vi "STAGE+mono+counter_edit14.vi"() -> ()   [LabVIEW 2017]
panel:
  out "XY Graph 2":cluster{dbl[], dbl[]}[](graph)
  out "XY Graph":cluster{dbl[], dbl[]}(graph)
  out "Slide":u8(slide) max=10 step=10 scale=0.0..10.0
  in  "?":enum32{"DELAY", "COUNTER", "MONO", "PLOT"}(tab)
  out "Final time [ps]":dbl
  out "Current time [ps]":dbl
  out "Initial time [ps]":dbl
  in  "Set this as t0":bool
  in  "Axis":i32=1
  in  "Motor ON":bool
  in  "Motor OFF":bool
  out "Current Position [mm]":dbl
  out "Final Position [mm]":dbl
  in  "Data Points":i32=100
  out "Current Point":i32
  in  "Step Size [um]":i32=10
  in  "Target [mm]":dbl format="%.3f"
  in  "Move":bool
  out "Initial position [mm]":dbl
  in  "GPIB address":string="23"
  in  "Count Mode":u16(ring) items=["A,B for Preset T", "A-B for Preset T", "A+B for Preset T", "A for Preset B"]
  in  "Trigger mode":u16(ring) items=["10 MHz"=0, "Input 2"=2, "Input T"=3]
  in  "Channel A Input":u16(ring)=1 items=["10 MHz", "Input 1"]
  in  "Channel B Input":u16(ring)=2 items=["Input 1"=1, "Input 2"=2]
  in  "Number of Measurements\n to take at one point/ Number of Periods":u16=1 min=1 max=2000 step=1
  in  "Time between measurements\n at one point (s)/Dwell Time":dbl=0.002 min=0.002 max=60.0 step=0.001
  in  "gate A mode (CW:0)":i16(slide) scale=0.0..2.0 scale format="%.2f"
  out "Counts":i32
  in  "Integrating time, 10^-7 sec":dbl=10000000.0
  out "Grating #":dbl
  out "Blaze angle":dbl
  out "Grooves/mm":dbl
  out "Mono port":T1(ring)
  out "Time delay":u32=450000 min=1
  in  "Step size":dbl=10.0 min=0.0
  in  "Scan to":i32=4000
  in  "Scan from":i32=2600
  out "Current wavelength":dbl
  in  "?":bool
  in  "Array":dbl[](array[numeric])
  out "Numeric":i32
  out "Numeric 2":i32
  out "Timeout 2":bool
  in  "?":bool
  out "Timeout":bool
  in  "Collect Data!":bool
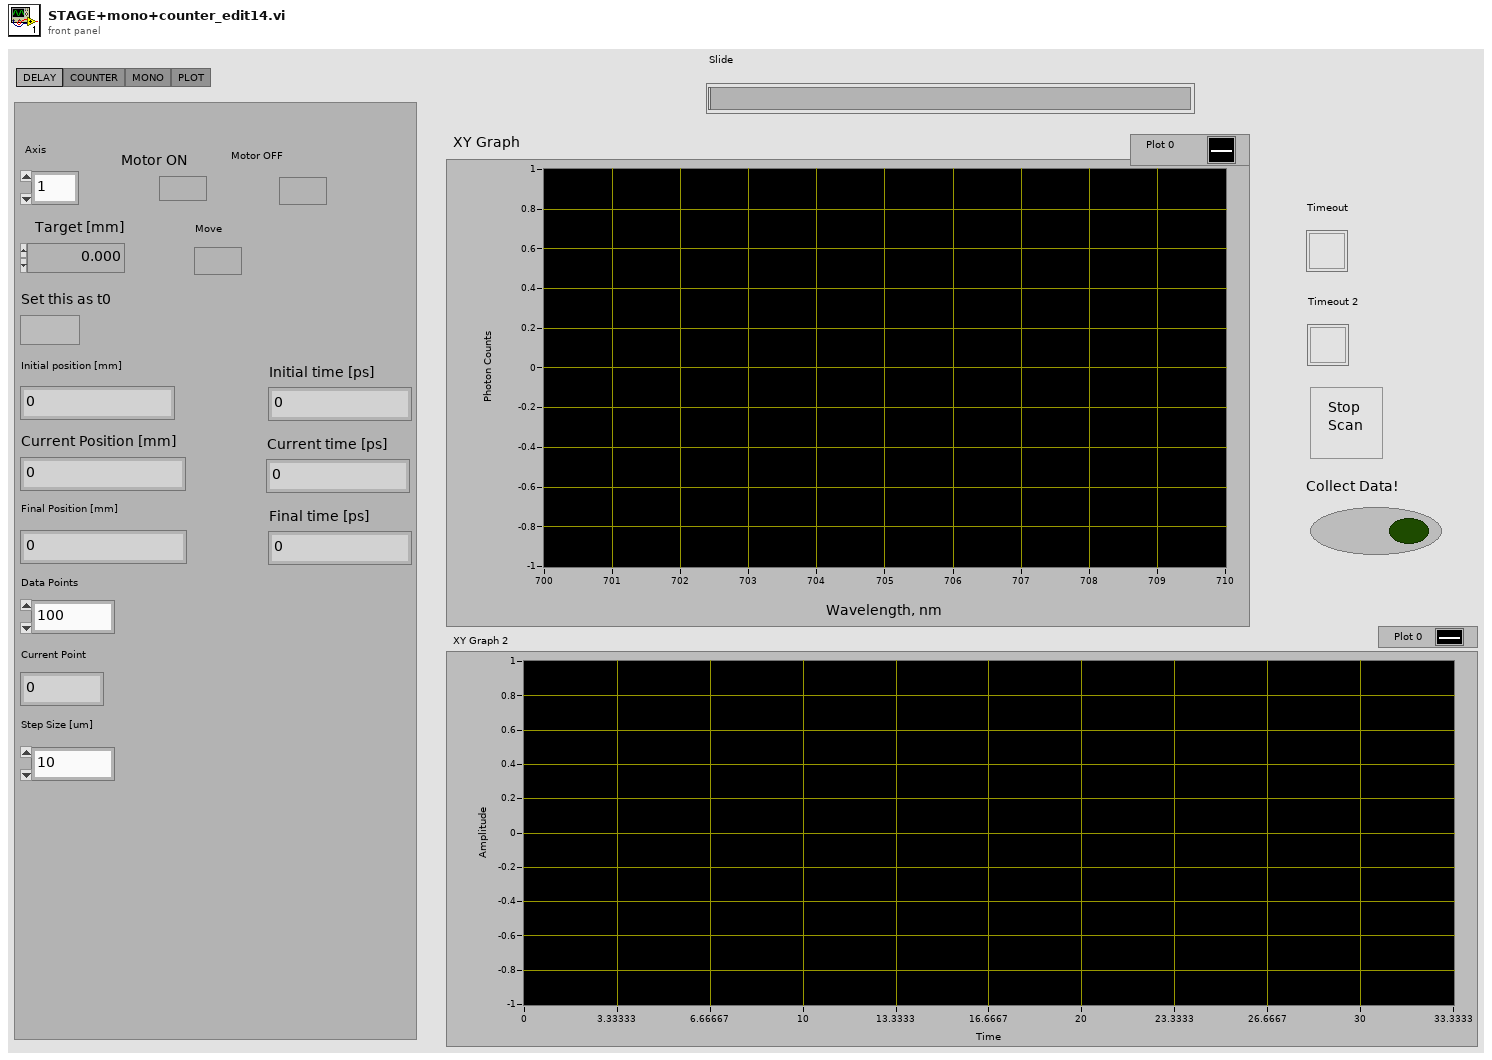
[diagram p1: front panel]
types:
  T1 = enum8{"COM 1", "COM 2", "COM 3", "COM 4", "COM 5", "COM 6", "COM 7", "COM 8", "COM 9"}
  T2 = cluster{"input XON/XOFF":bool, "input HW Handshake":bool, "input alt HW HShk":bool, "output XON/XOFF":bool, "output HW Handshake":bool, "output alt HW HShk":bool, "XOFF byte":u8, "XON byte":u8, "parity error byte":u16}
  T3 = enum16{"no parity", "odd parity", "even parity", "mark parity", "space parity"}
  T4 = cluster{"Y[0]":dbl, "Y[1]":dbl, "Y[2]":dbl, "Y[3]":dbl, "Y[4]":dbl, "Y[5]":dbl, "Y[6]":dbl, "Y[7]":dbl, "Y[8]":dbl}
  T5 = typedef "NI_Matrix.lvlib/RealMatrix.ctl" = dbl[][]
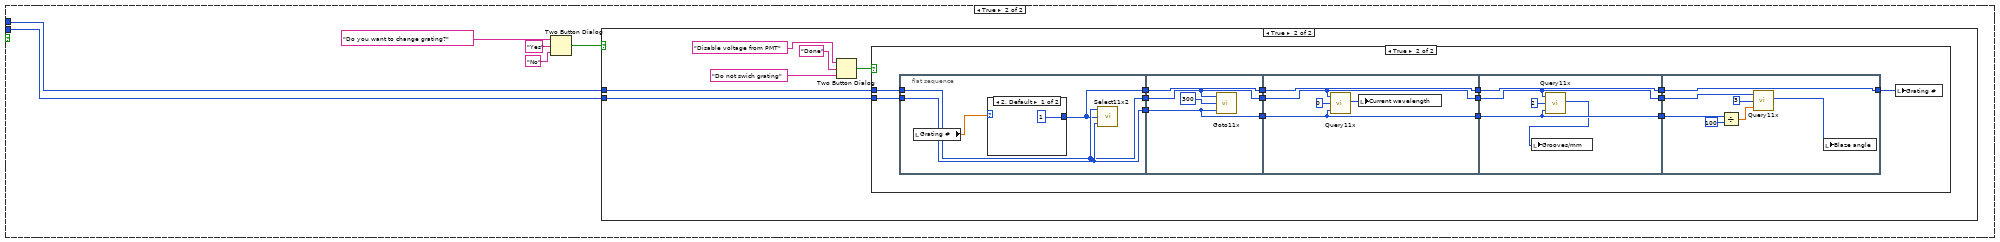
[diagram p2: hidden frame]
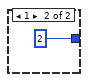
[diagram p5: hidden frame]
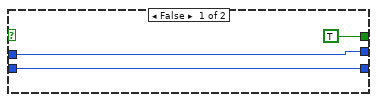
[diagram p6: hidden frame]
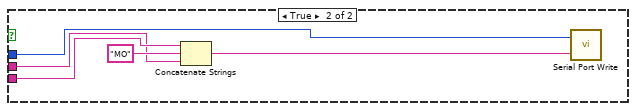
[diagram p7: hidden frame]
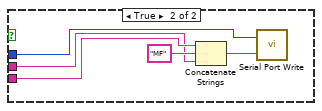
[diagram p8: hidden frame]
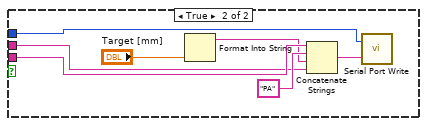
[diagram p9: hidden frame]
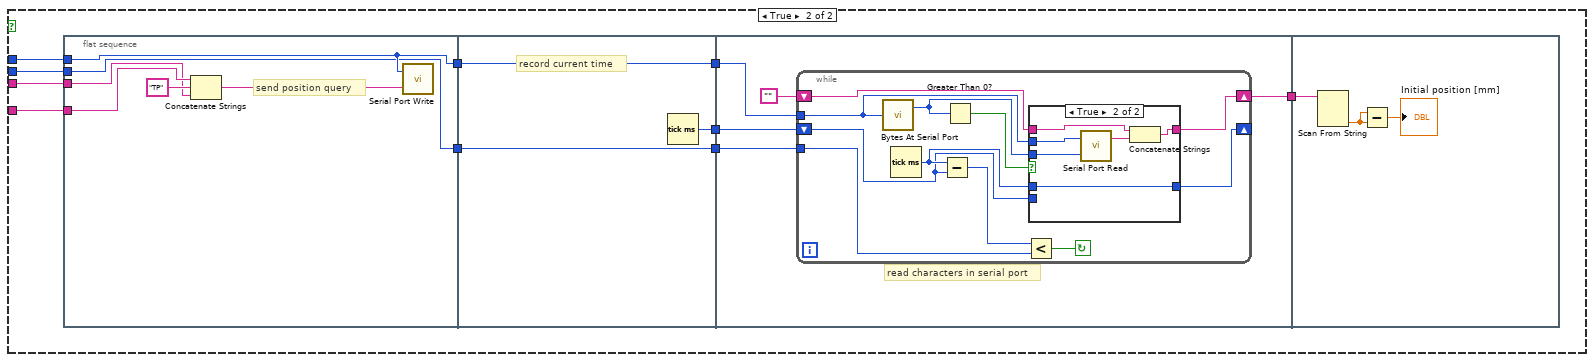
[diagram p10: hidden frame]
diagram:
  (unwired) FALSE
  w48 = u32 19200  # baud rate
  w47 = u16 8  # data bits
  w46 = enum16{"1 bit", "1.5 bits", "2 bits"}."1 bit"  # stop bits
  w50 = T3."no parity"  # parity
  w45 = 4  # 0=COM1 so n=COM(n+1)
  w49 = u16 1024  # buffer size
  n1 = flat-sequence {
    tunnel: ["Data Points"] -> w54
    tunnel: "Axis" -> [w76]
    tunnel: [w68] -> w53
    tunnel: [w76] -> w52
    tunnel: ["Step Size [um]"] -> w14
    tunnel: [w68] -> w13
    tunnel: ["Step Size [um]"] -> w12
    tunnel: ["Data Points"] -> w11
    tunnel: [w68] -> w10
    tunnel: [w67] -> w9
    tunnel: [w68] -> w7
    tunnel: [w67] -> w6
    tunnel: [w70] -> w5
    tunnel: [w60] -> w4
    tunnel: w54 -> [w138]
    tunnel: w53 -> [w137]
    tunnel: w52 -> [w136]
    tunnel: w45 -> [w132]
    tunnel: "GPIB address" -> [w131]
    tunnel: w16 -> [w130]
    tunnel: w15 -> [w129]
    tunnel: "GPIB address" -> [w128]
    tunnel: w14 -> [w115]
    tunnel: w13 -> [w113]
    tunnel: w12 -> [w112]
    tunnel: w11 -> [w110]
    tunnel: w10 -> [w103]
    tunnel: w9 -> [w102]
    tunnel: "Integrating time, 10^-7 sec" -> [w101]
    tunnel: w7 -> [w99]
    tunnel: w6 -> [w98]
    tunnel: w5 -> [w97]
    tunnel: w4 -> [w95]
    frame #0 {
      n2 = while {
        stop <- "Collect Data!" stop-if-true
        n3 = Multiply(x=1, y=1000) -> (x*y=w58:i32)
        n4 = Wait (ms)(milliseconds to wait=w58) -> ()  [unwired: 1 out]
      }
    }
    frame #1 {
      w61 = 1000000000000.0
      w66 = 1000
      w69 = 300000000
      w71 = 1000
      n5 = local read "Initial position [mm]"() -> (w68:dbl)
      n6 = Multiply(x="Step Size [um]", y="Data Points") -> (x*y=w75:i32)
      n7 = Divide(x="Step Size [um]", y=w71) -> (x/y=w70:dbl)
      n8 = Divide(x=w75, y=w71) -> (x/y=w74:dbl)
      n9 = Add(x=w68, y=w74) -> (x+y=w67:dbl)
      "Final Position [mm]" <- w67
      n10 = Divide(x=w68, y=w66) -> (x/y=w64:dbl)
      n11 = Divide(x=w67, y=w66) -> (x/y=w65:dbl)
      n12 = Divide(x=w64, y=w69) -> (x/y=w63:dbl)
      n13 = Divide(x=w65, y=w69) -> (x/y=w62:dbl)
      n14 = Multiply(x=w62, y=w61) -> (x*y=→"Final time [ps]":dbl)
      n15 = Multiply(x=w63, y=w61) -> (x*y=w60:dbl)
      "Initial time [ps]" <- w60
    }
    frame #2 {
      n16 = Increment(x=w110) -> (x+1=w111:i32)
      n17 = Divide(x=w115, y=1000.0) -> (x/y=w89:dbl)
      n18 = for {
        N: w111 -> [_]
        tunnel: w89 -> [w149]
        tunnel: w113 -> [w147]
        tunnel: [w140] -> w109 mode=indexing
        i -> [w148]
        # "distances"
        n19 = Multiply(x=w149, y=w148) -> (x*y=w146:dbl)
        n20 = Add(x=w147, y=w146) -> (x+y=w145:dbl)
        n21 = Divide(x=w145, y=1000) -> (x/y=w139:dbl)
        n22 = Divide(x=w139, y=300000000) -> (x/y=w142:dbl)
        n23 = Multiply(x=w142, y=1000000000000.0) -> (x*y=w140:dbl)
      }
      n24 = Multiply(x="Scan to", y=1) -> (x*y=w96:i32)
      n25 = Multiply(x=1, y="Scan from") -> (x*y=w85:i32)
      n26 = Divide(x=w89, y=1000.0) -> (x/y=w90:dbl)
      n27 = Subtract(x=w96, y=w85) -> (x-y=w123:i32)
      n28 = local read "Numeric 2"() -> (w78:i32)
      n29 = local read "Numeric"() -> (w77:i32)
      n30 = Divide(x=w123, y="Step size") -> (x/y=w122:dbl)
      n31 = Divide(x=w90, y=300000000) -> (x/y=w92:dbl)
      n32 = Multiply(x=w92, y=1000000000000.0) -> (x*y=w88:dbl)
      n33 = Build Array(w95) -> (w82:dbl[])
      n34 = Round Toward -Infinity(1:w122) -> (0:w121:dbl)
      n35 = Concatenate Strings("\r", "\n") -> (w133:string)
      n36 = Initialize Array(0, w77, w78) -> (w80:i32[][])
      n37 = Increment(x=w121) -> (x+1=w84:dbl)
      n38 = for {
        N: w138 -> [w197]
        tunnel: w137 -> [w224]
        tunnel: w112 -> [w220]
        tunnel: w136 -> [w217]
        tunnel: w133 -> [w214]
        tunnel: w132 -> [w215]
        tunnel: w131 -> [w213]
        tunnel: w130 -> [w210]
        tunnel: w129 -> [w212]
        tunnel: w128 -> [w211]
        tunnel: [w162] -> w118 mode=indexing
        tunnel: w85 -> [w205]
        tunnel: "Step size" -> [w204]
        tunnel: w121 -> [w203]
        tunnel: w103 -> [_]
        tunnel: w102 -> [_]
        tunnel: w101 -> [w202]
        tunnel: "Scan to" -> [w201]
        tunnel: "Scan from" -> [w200]
        tunnel: "Step size" -> [w171]
        tunnel: w99 -> [w192]
        tunnel: w98 -> [w190]
        tunnel: w97 -> [w193]
        tunnel: w88 -> [w180]
        shift-right: [w164] -> _
        shift-left: w82 -> [w174]
        shift-right: [w163] -> _
        shift-left: dbl[] [] ("Y") -> [w169]
        tunnel: w95 -> [w198]
        tunnel: "Scan from" -> [w172]
        tunnel: "Step size" -> [w173]
        shift-right: [w161] -> _
        shift-left: w82 -> [w167]
        shift-right: [w159] -> _
        shift-left: w80 -> [w158]
        i -> [w179]
        w191 = 1000
        w194 = 300000000
        n39 = To Time Stamp(1:w205) -> ()  [unwired: 1 out]
        n40 = property on="Slide" class="Slide (strict)"("Scale.Increment"=1, "Scale.Maximum"=w197, "Scale.Minimum"=0) -> ()  [unwired: 2 in, 2 out]
        n41 = stacked-sequence {
          tunnel: w210 -> [w344]
          tunnel: w211 -> [_]
          frame #0 {
            n42 = call <vilib>:"Close Serial Driver.vi"("port number"=w344) -> ()  [unwired: 1 out]
            n43 = GPIB Misc(0:"loc 23" ("command string")) -> ()  [unwired: 1 in, 3 out]
          }
        }
        n44 = Multiply(x=w180, y=w179) -> (x*y=w199:dbl)
        n45 = Divide(x=w192, y=w191) -> (x/y=w188:dbl)
        n46 = Divide(x=w193, y=w191) -> (x/y=w189:dbl)
        n47 = Divide(x=w190, y=w191) -> (x/y=w187:dbl)
        n48 = Number To Decimal String(number=w202) -> (decimal integer string=w208:string)  [unwired: 1 in]
        n49 = Build Array(w172) -> (w176:i32[])
        n50 = Add(x=1, y=w179) -> (x+y=→"Slide":i32)
        n51 = Divide(x=w220, y=1000) -> (x/y=w219:dbl)
        n52 = Divide(x=w188, y=w194) -> (x/y=w182:dbl)
        n53 = Divide(x=w189, y=w194) -> (x/y=w183:dbl)
        n54 = Divide(x=w187, y=w194) -> (x/y=w181:dbl)
        n55 = Add(x=w198, y=w199) -> (x+y=w168:dbl)
        n56 = Concatenate Strings("CP 2,", w208) -> (w206:string)
        n57 = flat-sequence {
          tunnel: w213 -> [w238]
          tunnel: w212 -> [w237]
          tunnel: w210 -> [w236]
          tunnel: w205 -> [w235]
          tunnel: w204 -> [w234]
          tunnel: w203 -> [w233]
          tunnel: w201 -> [w232]
          tunnel: w200 -> [w231]
          tunnel: w176 -> [w230]
          tunnel: dbl[] [] ("Y") -> [w229]
          tunnel: w173 -> [w228]
          tunnel: w172 -> [w227]
          tunnel: w171 -> [w226]
          tunnel: [w225] -> w170
          tunnel: w170 -> [w298]
          tunnel: w169 -> [w305]
          tunnel: [w298] -> w166
          tunnel: w165 -> [w302]
          tunnel: [w300] -> w164
          tunnel: [w299] -> w163
          tunnel: [w298] -> w162
          tunnel: w166 -> [w314]
          tunnel: [w307] -> w161
          tunnel: w160 -> [w308]
          tunnel: w158 -> [w311]
          tunnel: [w309] -> w159
          frame #0 {
            # "step size"
            n58 = while {
              tunnel: w236 -> [w270]
              tunnel: w237 -> [w269]
              tunnel: w238 -> [w265]
              tunnel: w235 -> [w263]
              tunnel: w234 -> [w262]
              tunnel: w233 -> [w261]
              tunnel: w232 -> [w245]
              tunnel: w231 -> [w246]
              tunnel: w226 -> [w247]
              tunnel: w228 -> [w259]
              shift-right: [w254] -> w225
              shift-left: w229 -> [w253]
              shift-right: [w248] -> _
              shift-left: w230 -> [w257]
              tunnel: w227 -> [w251]
              i -> [w260]
              stop <- w268 stop-if-true
              n59 = property on="XY Graph" class="XYGraph (strict)"("XScale.Increment"=w247, "XScale.Maximum"=w245, "XScale.Minimum"=w246) -> ()  [unwired: 2 in, 2 out]
              n60 = Multiply(x=w260, y=w262) -> (x*y=w271:dbl)
              n61 = Multiply(x=w260, y=w259) -> (x*y=w258:dbl)
              n62 = Greater Or Equal?(x=w260, y=w261) -> (x >= y?=w266:bool)
              n63 = Add(x=w258, y=w251) -> (x+y=w256:dbl)
              n64 = Add(x=w271, y=w263) -> (x+y=w264:dbl)
              n65 = Or(x="?", y=w266) -> (x .or. y?=w268:bool)
              n66 = flat-sequence {
                tunnel: w264 -> [w276]
                tunnel: w270 -> [w275]
                tunnel: w269 -> [w274]
                tunnel: w265 -> [w272]
                tunnel: [w275] -> w244
                tunnel: [w274] -> w243
                tunnel: [w272] -> w242
                tunnel: w244 -> [w283]
                tunnel: w243 -> [w282]
                tunnel: w242 -> [w277]
                tunnel: [w277] -> w241
                tunnel: w241 -> [w285]
                tunnel: [w285] -> w240
                tunnel: w240 -> [w286]
                tunnel: [w286] -> w239
                tunnel: [w292] -> w250
                tunnel: w239 -> [w293]
                frame #0 {
                  n67 = call "Goto11x.vi"("time delay"=w274, "WAVELENGTH"=w276, "port number"=w275) -> ("timeout"=w273:bool)  [unwired: 2 out]
                  n68 = local write "Timeout 2"(w273) -> ()
                }
                frame #1 {
                  # "set counter time in 10^-7 seconds in CW"
                  n69 = call "Query11x.vi"("port number"=w283, "QUERY"=0, "time delay"=w282) -> ("timeout"=w281:bool, "STATUS MESSAGE"=w280:u16)  [unwired: 2 out]
                  n70 = local write "Timeout 2"(w281) -> ()
                  n71 = Divide(x=w280, y=10) -> (x/y=w279:dbl)
                  n72 = local write "Current wavelength"(w279) -> ()
                }
                frame #2 {
                  n73 = call "Start.vi"("GPIB Address"=w285) -> ()  [unwired: 9 in]
                }
                frame #3 {
                  # "Wait for Scan to Finish"
                  n74 = for {
                    N: 1 -> [_]
                    tunnel: w286 -> [w288]
                    n75 = while {
                      tunnel: w288 -> [w289]
                      stop <- w291 stop-if-true
                      n76 = call "ScanDone.vi"("Wait (ms)"=1000, "GPIB Address"=w289) -> ("Scan Finished?"=w291:bool)
                    }
                  }
                }
                frame #4 {
                  n77 = call "Read Data.vi"("Channel Number"=0, "GPIB Address"=w293, "Number of Datapoints"=1) -> ("Data"=w294:i32[])
                  n78 = Index Array(array=w294, index=0) -> (element=w292:i32)
                  "Counts" <- w292
                }
              }
              n79 = Build Array (concatenate)(w257, w256) -> (w255:dbl[])
              n80 = Build Array (concatenate)(w253, w250) -> (w252:dbl[])
              n81 = Bundle(w255, w252) -> (w249:cluster{dbl[], dbl[]})  [unwired: 1 in]
              "XY Graph" <- w249
              n82 = Unbundle(w249) -> (w248:dbl[], w254:dbl[])
            }
          }
          frame #1 {
            n83 = Array To Cluster(array=w298) -> (cluster=w306:T4)
            n84 = Unbundle By Name(w306) -> ("Y[5]"=w304:dbl)  [unwired: 10 out]
            n85 = Build Array (concatenate)(w305, w304) -> (w303:dbl[])
            n86 = Bundle(w302, w303) -> (w301:cluster{dbl[], dbl[]})  [unwired: 1 in]
            n87 = Unbundle(w301) -> (w300:dbl[], w299:dbl[])
          }
          frame #2 {
            n88 = Array Size(array="Array") -> (size(s)=w312:i32)
            n89 = flat-sequence {
              tunnel: w314 -> [w319]
              tunnel: "Array" -> [w318]
              tunnel: w312 -> [w317]
              tunnel: [w315] -> w310
              tunnel: w311 -> [w336]
              tunnel: w310 -> [w335]
              tunnel: [w333] -> w309
              tunnel: w308 -> [w332]
              tunnel: [w331] -> w307
              frame #0 {
                n90 = for {
                  N: w317 -> [w321]
                  tunnel: w318 -> [w329]
                  tunnel: w319 -> [w323]
                  tunnel: [w320] -> w316
                  i -> [w328]
                  n91 = local read "Scan from"() -> (w326:i32)
                  n92 = Index Array(array=w329, index=w328) -> (element=w327:dbl)
                  n93 = local read "Step size"() -> (w324:dbl)
                  n94 = Subtract(x=w327, y=w326) -> (x-y=w325:dbl)
                  n95 = Divide(x=w325, y=w324) -> (x/y=w322:dbl)
                  n96 = Index Array(array=w323, index=w322) -> (element=w320:dbl)
                  "Numeric" <- w321
                }
                n97 = Build Array(w316) -> (w315:dbl[])
              }
              frame #1 {
                n98 = local read "Numeric"() -> (w334:i32)
                n99 = Build Array (concatenate)(w336, w335) -> (w333:dbl[][])
                n100 = for {
                  N: w334 -> [_]
                  tunnel: w333 -> [w342]
                  tunnel: w332 -> [w340]
                  tunnel: [w339] -> w331
                  tunnel: [w337] -> w330 mode=indexing
                  i -> [w341]
                  n101 = Index Array(array=w342, index (row)=w341) -> (element=w338:dbl[])  [unwired: 1 in]
                  n102 = Bundle(w340, w338) -> (w337:cluster{dbl[], dbl[]})  [unwired: 1 in]
                  n103 = Unbundle(w337) -> (w339:dbl[])  [unwired: 1 out]
                }
                "XY Graph 2" <- w330
              }
            }
          }
        }
        n104 = Multiply(x=w219, y=w179) -> (x*y=w223:dbl)
        n105 = Multiply(x=w182, y=1000000000000.0) -> (x*y=w156:dbl)
        n106 = Multiply(x=w183, y=1000000000000.0) -> (x*y=w157:dbl)
        n107 = Multiply(x=w181, y=1000000000000.0) -> (x*y=w155:dbl)
        n108 = Build Array (concatenate)(w167, w168) -> (w160:dbl[])
        n109 = Build Array (concatenate)(w174, w168) -> (w165:dbl[])
        n110 = property on="XY Graph 2" class="XYGraph (strict)"("XScale.Increment"=w157, "XScale.Maximum"=w155, "XScale.Minimum"=w156) -> ()  [unwired: 2 in, 2 out]
        n111 = Add(x=w224, y=w223) -> (x+y=w222:dbl)
        n112 = Format Into String(w217) -> (resulting string=w216:string)  [unwired: 3 in, 1 out]
        n113 = GPIB Write(0:w213, 1:w206, 2:i16 5 ("mode (0)")) -> ()  [unwired: 2 in, 2 out]
        n114 = flat-sequence {
          tunnel: w222 -> [w347]
          tunnel: [w347] -> w218
          tunnel: w214 -> [w349]
          tunnel: w216 -> [w348]
          tunnel: w215 -> [w345]
          tunnel: w218 -> [w358]
          frame #0 {
            n115 = Format Into String(w347) -> (resulting string=w346:string)  [unwired: 3 in, 1 out]
            n116 = Wait (ms)(milliseconds to wait=u32 100) -> ()  [unwired: 1 out]
            n117 = Concatenate Strings(w348, "PA" ("Substring"), w346, w349) -> (w351:string)
            n118 = call <vilib>:"Serial Port Write.vi"("string to write"=w351, "port number"=w345) -> ()  [unwired: 1 out]
          }
          frame #1 {
            n119 = Divide(x=w358, y=1000) -> (x/y=w356:dbl)
            n120 = Wait (ms)(milliseconds to wait=u32 1000) -> ()  [unwired: 1 out]
            n121 = Divide(x=w356, y=300000000) -> (x/y=w355:dbl)
            n122 = Multiply(x=w355, y=1000000000000.0) -> (x*y=→"Current time [ps]":dbl)
            "Current Position [mm]" <- w358
          }
        }
        "Current Point" <- w179
        "Numeric 2" <- w197
      }
      n123 = for {
        N: w84 -> [_]
        tunnel: "Step size" -> [w154]
        tunnel: w85 -> [w152]
        tunnel: [w150] -> w83 mode=indexing
        i -> [w153]
        # "wavelengths"
        n124 = Multiply(x=w154, y=w153) -> (x*y=w151:dbl)
        n125 = Add(x=w152, y=w151) -> (x+y=w150:dbl)
      }
      n126 = Build Array (concatenate)(0, w109) -> (w106:dbl[])
      n127 = Build Array(w83) -> (w119:dbl[][])
      n128 = Transpose Matrix(1:w118) -> (0:w116:dbl[][])
      n129 = Transpose Matrix(1:w119) -> (0:w117:dbl[][])
      n130 = Build Array (concatenate)(w117, w116) -> (w105:T5)
      n131 = Insert Into Array(array=w105, index (row)=0, new element=w106) -> (w104:T5)  [unwired: 1 in]
      n132 = Array To Spreadsheet String(delimiter (Tab)=",", array=w104, 3:"%f" ("format string")) -> (spreadsheet string=w120:string)
      n133 = Write to Text File(text=w120) -> ()  [unwired: 3 in, 3 out]
    }
  }
  n134 = flat-sequence {
    tunnel: [w362] -> w30
    tunnel: [w361] -> w29
    frame #0 {
      n135 = call "CM Com Read ini.vi"() -> ("Mono port"=w361:T1, "time delay1"=w362:u32)  [unwired: 7 in]
    }
  }
  n136 = call <vilib>:"Serial Port Init.vi"("flow control etc."=T2 {"input XON/XOFF"=FALSE, "input HW Handshake"=FALSE, "input alt HW HShk"=FALSE, "output XON/XOFF"=FALSE, "output HW Handshake"=FALSE, "output alt HW HShk"=FALSE, "XOFF byte"=13, "XON byte"=11, "parity error byte"=0}, "parity"=w50, "buffer size"=w49, "stop bits"=w46, "data bits"=w47, "baud rate"=w48, "port number"=w45) -> ("error code"=w44:i32)
  n137 = call "CM Serial Port Setup.vi"("COM port"=w29, "time delay"=w30) -> ("time delay1"=w25:u32, "DK port Out"=w26:T1, "error code"=w28:i32)  [unwired: 7 in]
  n138 = Concatenate Strings("\r", "\n") -> (w40:string)
  n139 = Equal To 0?(x=w28) -> (x = 0?=w27:bool)
  n140 = while {
    tunnel: w45 -> [w377]
    tunnel: w40 -> [w378]
    tunnel: w44 -> [_]
    tunnel: "Axis" -> [w375]
    stop <- TRUE continue-if-true
    w376 = u32 200  # timeout
    n141 = Format Into String(w375) -> (resulting string=w379:string)  [unwired: 3 in, 1 out]
    n142 = flat-sequence {
      tunnel: w379 -> [w384]
      tunnel: w378 -> [w383]
      tunnel: w377 -> [w385]
      tunnel: w376 -> [w382]
      tunnel: [w384] -> w374
      tunnel: [w383] -> w373
      tunnel: [w385] -> w372
      tunnel: [w382] -> w371
      tunnel: w374 -> [w395]
      tunnel: w373 -> [w394]
      tunnel: w372 -> [w396]
      tunnel: w371 -> [w392]
      tunnel: [w395] -> w370
      tunnel: [w394] -> w369
      tunnel: [w396] -> w368
      tunnel: [w392] -> w367
      tunnel: w370 -> [w405]
      tunnel: w369 -> [w404]
      tunnel: w368 -> [w406]
      tunnel: w367 -> [w402]
      tunnel: [w405] -> w366
      tunnel: [w404] -> w365
      tunnel: [w406] -> w364
      tunnel: [w402] -> w363
      tunnel: w366 -> [w418]
      tunnel: w365 -> [w415]
      tunnel: w364 -> [w417]
      tunnel: w363 -> [w416]
      frame #0 {
        n143 = case shown="False" "Motor ON" {
          tunnel: w385 -> [_ w391]
          tunnel: w384 -> [_ w388]
          tunnel: w383 -> [_ w387]
          frame False {
          }
          frame True {
            n144 = Concatenate Strings(w388, "MO" ("Substring"), w387) -> (w389:string)
            n145 = call <vilib>:"Serial Port Write.vi"("string to write"=w389, "port number"=w391) -> ()  [unwired: 1 out]
          }
        }
      }
      frame #1 {
        n146 = case shown="False" "Motor OFF" {
          tunnel: w396 -> [_ w401]
          tunnel: w395 -> [_ w398]
          tunnel: w394 -> [_ w397]
          frame False {
          }
          frame True {
            n147 = Concatenate Strings(w398, "MF" ("Substring"), w397) -> (w399:string)
            n148 = call <vilib>:"Serial Port Write.vi"("string to write"=w399, "port number"=w401) -> ()  [unwired: 1 out]
          }
        }
      }
      frame #2 {
        n149 = case shown="False" "Move" {
          tunnel: w406 -> [_ w413]
          tunnel: w405 -> [_ w410]
          tunnel: w404 -> [_ w409]
          frame False {
          }
          frame True {
            n150 = Format Into String("Target [mm]") -> (resulting string=w407:string)  [unwired: 3 in, 1 out]
            n151 = Concatenate Strings(w410, "PA" ("Substring"), w407, w409) -> (w411:string)
            n152 = call <vilib>:"Serial Port Write.vi"("string to write"=w411, "port number"=w413) -> ()  [unwired: 1 out]
          }
        }
      }
      frame #3 {
        n153 = case shown="False" "Set this as t0" {
          tunnel: w418 -> [_ w428]
          tunnel: w417 -> [_ w427]
          tunnel: w416 -> [_ w426]
          tunnel: w415 -> [_ w425]
          frame False {
          }
          frame True {
            n154 = flat-sequence {
              tunnel: w428 -> [w432]
              tunnel: w427 -> [w431]
              tunnel: [w431] -> w424
              tunnel: w426 -> [w429]
              tunnel: [w429] -> w423
              tunnel: w425 -> [w430]
              tunnel: w424 -> [w436]
              tunnel: [w436] -> w422
              tunnel: w423 -> [w435]
              tunnel: [w435] -> w421
              tunnel: [w437] -> w420
              tunnel: w422 -> [w442]
              tunnel: w421 -> [w440]
              tunnel: w420 -> [w439]
              tunnel: [w438] -> w419
              tunnel: w419 -> [w464]
              frame #0 {
                # "send position query"
                n155 = Concatenate Strings(w432, "TP" ("Substring"), w430) -> (w433:string)
                n156 = call <vilib>:"Serial Port Write.vi"("string to write"=w433, "port number"=w431) -> ()  [unwired: 1 out]
              }
              frame #1 {
                # "record current time"
                n157 = Tick Count (ms)() -> (millisecond timer value=w437:u32)
              }
              frame #2 {
                # "read characters in serial port"
                n158 = while {
                  shift-left: w439 -> [w443]
                  shift-right: [w444] -> _
                  tunnel: w440 -> [w447]
                  shift-left: "" -> [w450]
                  shift-right: [w449] -> w438
                  tunnel: w442 -> [w451]
                  stop <- w446 continue-if-true
                  n159 = call <vilib>:"Bytes At Serial Port.vi"("port number"=w451) -> ("byte count"=w452:u32)  [unwired: 1 out]
                  n160 = Tick Count (ms)() -> (millisecond timer value=w445:u32)
                  n161 = Subtract(x=w445, y=w443) -> (x-y=w448:u32)
                  n162 = Greater Than 0?(x=w452) -> (x > 0?=w453:bool)
                  n163 = Less?(x=w448, y=w447) -> (x < y?=w446:bool)
                  n164 = case shown="True" w453 {
                    tunnel: w452 -> [_ w461]
                    tunnel: w451 -> [_ w460]
                    tunnel: w450 -> [w455 w458]
                    tunnel: [w455 w457] -> w449
                    tunnel: [w454 w456] -> w444
                    tunnel: w445 -> [_ w456]
                    tunnel: w443 -> [w454 _]
                    frame False {
                    }
                    frame True {
                      n165 = call <vilib>:"Serial Port Read.vi"("requested byte count"=w461, "port number"=w460) -> ("string read"=w459:string)  [unwired: 1 out]
                      n166 = Concatenate Strings(w458, w459) -> (w457:string)
                    }
                  }
                }
              }
              frame #3 {
                n167 = Scan From String(input string=w464) -> (output 1=w462:dbl)  [unwired: 4 in, 3 out]
                n168 = Subtract(x=w462, y=w462) -> (x-y=→"Initial position [mm]":dbl)
              }
            }
          }
        }
      }
    }
    n169 = Wait Until Next ms Multiple(millisecond multiple=u32 50) -> ()  [unwired: 1 out]
  }
  n170 = case shown="True" w27 {
    tunnel: w26 -> [w467 w470]
    tunnel: w25 -> [w466 w469]
    tunnel: [w467 w470] -> w16
    tunnel: [w466 w469] -> w15
    tunnel: [TRUE FALSE] -> w24
    frame False {
    }
    frame True {
      n171 = call "CM Com Write ini.vi"("time delay1"=w470, "Mono port"=w469) -> ()  [unwired: 7 in]
      n172 = local write "Mono port"(w470) -> ()
      n173 = local write "Time delay"(w469) -> ()
    }
  }
  n174 = flat-sequence {
    tunnel: w15 -> [w476]
    tunnel: [w476] -> w39
    tunnel: w16 -> [w478]
    tunnel: [w478] -> w38
    tunnel: w24 -> [w474]
    tunnel: [w474] -> w37
    tunnel: w39 -> [w482]
    tunnel: [w482] -> w36
    tunnel: w38 -> [w483]
    tunnel: [w483] -> w35
    tunnel: w37 -> [w480]
    tunnel: [w480] -> w34
    tunnel: w36 -> [w491]
    tunnel: [w491] -> w33
    tunnel: w35 -> [w488]
    tunnel: [w488] -> w32
    tunnel: w34 -> [w486]
    tunnel: [w486] -> w31
    tunnel: w33 -> [w494]
    tunnel: w32 -> [w493]
    tunnel: w31 -> [_]
    frame #0 {
      n175 = call "Query11x.vi"("port number"=w478, "QUERY"=u16 0, "time delay"=w476) -> ("timeout"=w475:bool, "STATUS MESSAGE"=w473:u16)  [unwired: 2 out]
      n176 = local write "Timeout"(w475) -> ()
      n177 = Divide(x=w473, y=10 ("Numeric")) -> (x/y=→"Current wavelength":dbl)
    }
    frame #1 {
      n178 = call "Query11x.vi"("port number"=w483, "QUERY"=u16 2, "time delay"=w482) -> ("timeout"=w481:bool, "STATUS MESSAGE"=→"Grooves/mm":u16)  [unwired: 2 out]
      n179 = local write "Timeout"(w481) -> ()
    }
    frame #2 {
      n180 = Divide(x=w491, y=i16 100 ("device (1)")) -> (x/y=w489:dbl)
      n181 = call "Query11x.vi"("port number"=w488, "QUERY"=u16 3, "time delay"=w489) -> ("timeout"=w487:bool, "STATUS MESSAGE"=→"Blaze angle":u16)  [unwired: 2 out]
      n182 = local write "Timeout"(w487) -> ()
    }
    frame #3 {
      n183 = Divide(x=w494, y=i16 100 ("device (1)")) -> (x/y=w497:dbl)
      n184 = call "Query11x.vi"("port number"=w493, "QUERY"=u16 4, "time delay"=w497) -> ("timeout"=w496:bool, "STATUS MESSAGE"=→"Grating #":u16)  [unwired: 2 out]
      n185 = local write "Timeout"(w496) -> ()
    }
  }
  n186 = case shown="False" "?" {
    tunnel: w15 -> [_ w501]
    tunnel: w16 -> [_ w500]
    frame False {
    }
    frame True {
      n187 = Two Button Dialog(message="Do you want to change grating?", 1:"No" ("F button name (\"Cancel\")"), 2:"Yes" ("T button name (\"OK\")")) -> (T button?=w502:bool)
      n188 = case shown="True" w502 {
        tunnel: w501 -> [_ w507]
        tunnel: w500 -> [_ w506]
        frame False {
        }
        frame True {
          n189 = Two Button Dialog(message="Disable voltage from PMT", 1:"Do not swich grating" ("F button name (\"Cancel\")"), 2:"Done" ("T button name (\"OK\")")) -> (T button?=w508:bool)
          n190 = case shown="True" w508 {
            tunnel: w507 -> [_ w526]
            tunnel: w506 -> [_ w525]
            frame False {
            }
            frame True {
              n191 = flat-sequence {
                tunnel: w526 -> [w530]
                tunnel: [w530] -> w523
                tunnel: w525 -> [w529]
                tunnel: [w529] -> w522
                tunnel: [w527] -> w521
                tunnel: w523 -> [w534]
                tunnel: [w534] -> w520
                tunnel: w522 -> [w535]
                tunnel: [w535] -> w519
                tunnel: w521 -> [w533]
                tunnel: [w533] -> w518
                tunnel: w520 -> [w541]
                tunnel: [w541] -> w517
                tunnel: w519 -> [w540]
                tunnel: [w540] -> w516
                tunnel: w518 -> [w538]
                tunnel: [w538] -> w515
                tunnel: w517 -> [w544]
                tunnel: [w544] -> w514
                tunnel: w516 -> [w545]
                tunnel: [w545] -> w513
                tunnel: w515 -> [w543]
                tunnel: [w543] -> w512
                tunnel: w514 -> [w549]
                tunnel: w513 -> [w550]
                tunnel: [w548] -> w524
                tunnel: w512 -> [w548]
                frame #0 {
                  n192 = local read "Grating #"() -> (w528:dbl)
                  n193 = case shown="2, Default" w528 {
                    tunnel: [1 2] -> w527
                    frame 2, Default {
                    }
                    frame 1 {
                    }
                  }
                  n194 = call "Select11x2.vi"("time delay"=w530, "NEW GRT?"=w527, "port number"=w529) -> ()  [unwired: 3 out]
                }
                frame #1 {
                  n195 = call "Goto11x.vi"("time delay"=w534, "WAVELENGTH"=u16 300, "port number"=w535) -> ()  [unwired: 3 out]
                }
                frame #2 {
                  n196 = call "Query11x.vi"("port number"=w540, "QUERY"=u16 0, "time delay"=w541) -> ("STATUS MESSAGE"=w537:u16)  [unwired: 3 out]
                  n197 = local write "Current wavelength"(w537) -> ()
                }
                frame #3 {
                  n198 = call "Query11x.vi"("port number"=w545, "QUERY"=u16 2, "time delay"=w544) -> ("STATUS MESSAGE"=w542:u16)  [unwired: 3 out]
                  n199 = local write "Grooves/mm"(w542) -> ()
                }
                frame #4 {
                  n200 = Divide(x=w549, y=i16 100 ("device (1)")) -> (x/y=w551:dbl)
                  n201 = call "Query11x.vi"("port number"=w550, "QUERY"=u16 3, "time delay"=w551) -> ("STATUS MESSAGE"=w547:u16)  [unwired: 3 out]
                  n202 = local write "Blaze angle"(w547) -> ()
                }
              }
              n203 = local write "Grating #"(w524) -> ()
            }
          }
        }
      }
    }
  }
  n204 = call "Configure.vi"("Dwell Time (s)"="Time between measurements\n at one point (s)/Dwell Time", "Channel T Input"="Trigger mode", "Channel B Input"="Channel B Input", "Channel A Input"="Channel A Input", "Integrating time, 10^-7 sec"="Integrating time, 10^-7 sec", "gate mode (CW:0)"="gate A mode (CW:0)", "Scan End Mode"=FALSE, "Number of Periods"="Number of Measurements\n to take at one point/ Number of Periods", "Count Mode"="Count Mode", "GPIB Address"="GPIB address") -> ()
  "Mono port" <- w29
  "Time delay" <- w30
